vi "generateTimeVector.vi"(2 "sampling time":dbl, 3 "record length":i16) -> (0 "time vector":dbl[](array[numeric]))   [LabVIEW 2010]
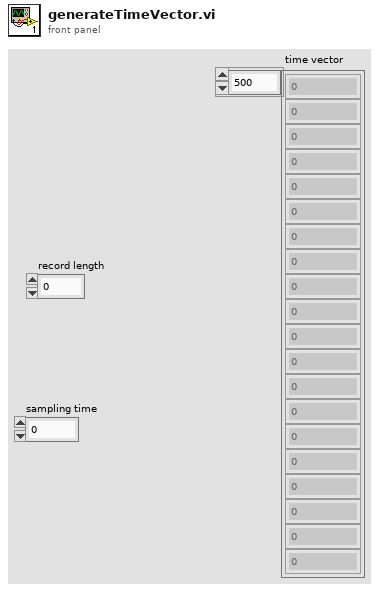
[diagram p1: front panel]
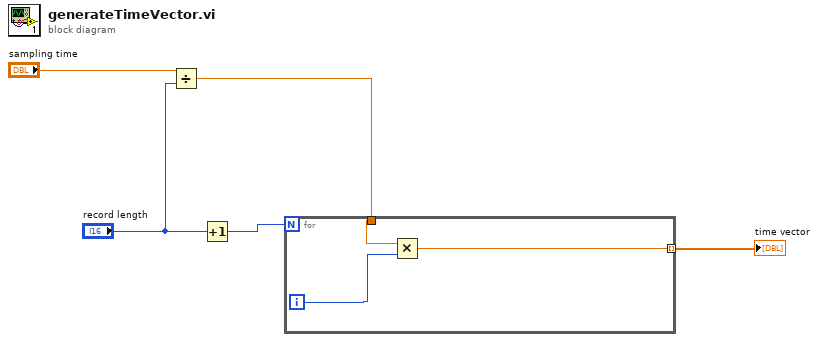
[diagram p0: block diagram]
diagram:
  n1 = Divide(x="sampling time", y="record length") -> (x/y=w4:dbl)
  n2 = Increment(x="record length") -> (x+1=w2:i16)
  n3 = for {
    N: w2 -> [_]
    tunnel: w4 -> [w8]
    tunnel: [w7] -> w3 mode=indexing
    i -> [w6]
    n4 = Multiply(x=w8, y=w6) -> (x*y=w7:dbl)
  }
  "time vector" <- w3
